vi "Subscr.Process Subscription Request.vi"(6 "Disable(Data2)":variant, 8 "error in (no error)":errorcluster, 9 "Request Info (Data1)":variant, 11 "Subscription in":refnum<class "Subscription.lvclass">) -> (0 "error out":errorcluster, 1 "SubScrReq":T1[](array[typedef]), 3 "Subscription out":refnum<class "Subscription.lvclass">)   [LabVIEW 2024, in "EQMF.lvlib" / "Subscription.lvlib" / "Subscription.lvclass"]
uses:
  Subscription.lvclass
  Subscr.Subscription Request Info.ctl
  Queues/Q.Element.ctl
  Subscription.lvclass/Subscription.ctl
  Queues/Queue Utils.lvlib
  Subscription.lvlib
panel:
  # "(For Ver/Debug)"
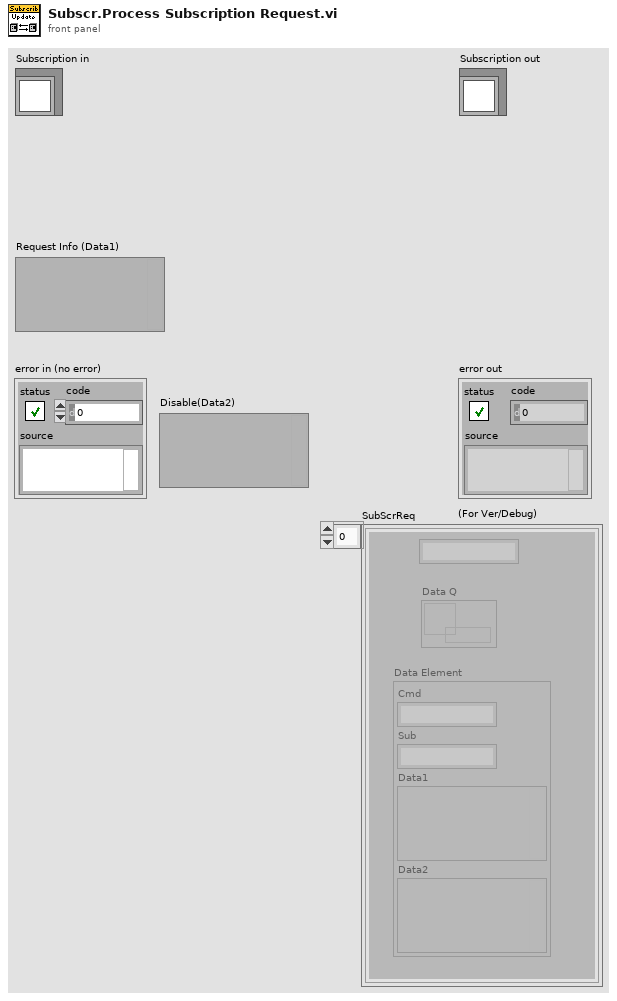
[diagram p1: front panel]
types:
  T1 = typedef "EQMF.lvlib/Subscription.lvlib/Subscr.Subscription Request Info.ctl" = cluster{"Name":string, "Data Q":refnum<queue>, "Data Element":T2}
  T2 = typedef "EQMF.lvlib/Queue Utils.lvlib/Q.Element.ctl" = cluster{"Cmd":string, "Sub":string, "Data1":variant, "Data2":variant}
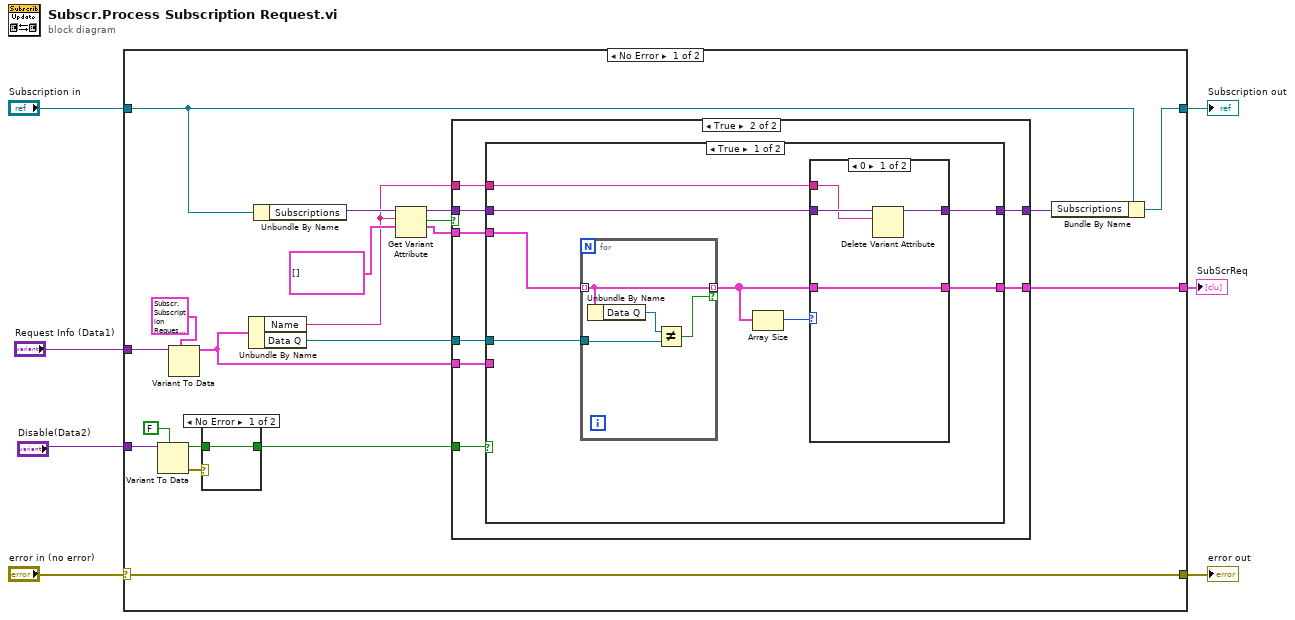
[diagram p0: block diagram]
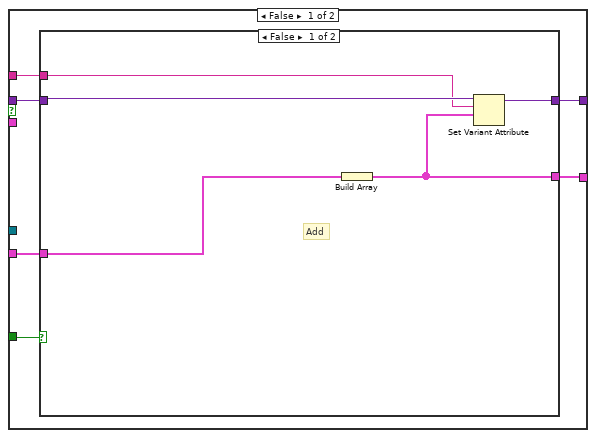
[diagram p2: hidden frame]
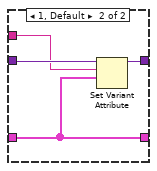
[diagram p4: hidden frame]
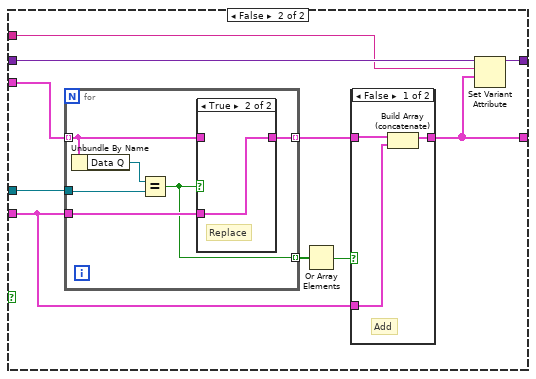
[diagram p5: hidden frame]
diagram:
  n1 = case shown="No Error" "error in (no error)" {
    selector: "error in (no error)" -> [w27 w92]
    tunnel: [w27 w92] -> w6
    tunnel: [w12 w91] -> w4
    tunnel: "Subscription in" -> [w11 w91]
    tunnel: "Request Info (Data1)" -> [w26 _]
    tunnel: "Disable(Data2)" -> [w24 _]
    tunnel: [w9 _] -> w1
    frame No Error {
      n2 = Variant To Data(type=FALSE, Variant=w24) -> (data=w21:bool, error out=w22:errorcluster)  [unwired: 1 in]
      n3 = Variant To Data(type=T1 {"Name"="", "Data Q"=refnum, "Data Element"={"Cmd"="", "Sub"="", "Data1"=variant, "Data2"=variant}} ("Event Destination"), Variant=w26) -> (data=w10:T1)  [unwired: 1 in, 1 out]
      n4 = case shown="No Error" w22 {
        tunnel: w21 -> [w90 _]
        tunnel: [w90 _] -> w14
        frame No Error {
        }
        frame Error {
        }
      }
      n5 = Unbundle By Name(w10) -> ("Name"=w8:string, "Data Q"=w15:refnum<queue>)
      n6 = Unbundle By Name(w11) -> ("Subscriptions"=w20:variant)
      n7 = Get Variant Attribute(Variant=w20, name=w8, default value (empty Variant)=T1[] []) -> (duplicate Variant=w17:variant, found=w18:bool, value=w16:T1[])  [unwired: 1 in, 1 out]
      n8 = case shown="True" w18 {
        tunnel: w17 -> [w32 w47]
        tunnel: w16 -> [_ w46]
        tunnel: w15 -> [_ w44]
        tunnel: w14 -> [w33 w45]
        tunnel: w8 -> [w30 w43]
        tunnel: [w31 w42] -> w13
        tunnel: w10 -> [w29 w41]
        tunnel: [w28 w40] -> w9
        frame False {
          n9 = case shown="False" w33 {
            tunnel: w32 -> [w37 w39]
            tunnel: [w38 w39] -> w31
            tunnel: w30 -> [w36 _]
            tunnel: w29 -> [w35 _]
            tunnel: [w34 _] -> w28
            frame False {
              # "Add"
              n10 = Build Array(w35) -> (w34:T1[])
              n11 = Set Variant Attribute(Variant=w37, name=w36, value=w34) -> (Variant out=w38:variant)  [unwired: 1 in, 2 out]
            }
            frame True {
              # "Do nothing.\nNo subscription to disable"
            }
          }
        }
        frame True {
          n12 = case shown="True" w45 {
            tunnel: w47 -> [w53 w75]
            tunnel: w46 -> [w55 w77]
            tunnel: w44 -> [w54 w76]
            tunnel: w43 -> [w51 w74]
            tunnel: [w50 w73] -> w42
            tunnel: w41 -> [_ w69]
            tunnel: [w48 w68] -> w40
            frame True {
              n13 = for {
                tunnel: w55 -> [w67] mode=indexing
                tunnel: w54 -> [w65]
                tunnel: [w67] -> w49 mode=indexing if=w64
                n14 = Unbundle By Name(w67) -> ("Data Q"=w66:refnum<queue>)
                n15 = Not Equal?(x=w66, y=w65) -> (x != y?=w64:bool)
              }
              n16 = Array Size(array=w49) -> (size(s)=w52:i32)
              n17 = case shown="0" w52 {
                tunnel: w53 -> [w59 w62]
                tunnel: w51 -> [w58 w61]
                tunnel: [w57 w63] -> w50
                tunnel: w49 -> [w56 w60]
                tunnel: [w56 w60] -> w48
                frame 0 {
                  n18 = Delete Variant Attribute(6:w58, 7:w59) -> (3:w57:variant)  [unwired: 1 in, 2 out]
                }
                frame 1, Default {
                  n19 = Set Variant Attribute(Variant=w62, name=w61, value=w60) -> (Variant out=w63:variant)  [unwired: 1 in, 2 out]
                }
              }
            }
            frame False {
              n20 = for {
                tunnel: w77 -> [w85] mode=indexing
                tunnel: w76 -> [w86]
                tunnel: [w83] -> w71 mode=indexing
                tunnel: w69 -> [w84]
                tunnel: [w82] -> w72 mode=indexing
                n21 = Unbundle By Name(w85) -> ("Data Q"=w87:refnum<queue>)
                n22 = Equal?(x=w87, y=w86) -> (x = y?=w82:bool)
                n23 = case shown="True" w82 {
                  tunnel: w85 -> [w88 _]
                  tunnel: w84 -> [_ w89]
                  tunnel: [w88 w89] -> w83
                  frame False {
                  }
                  frame True {
                    # "Replace"
                  }
                }
              }
              n24 = Or Array Elements(Boolean array=w72) -> (logical OR=w70:bool)
              n25 = case shown="False" w70 {
                tunnel: w71 -> [w80 w81]
                tunnel: w69 -> [w78 _]
                tunnel: [w79 w81] -> w68
                frame False {
                  # "Add"
                  n26 = Build Array (concatenate)(w80, w78) -> (w79:T1[])
                }
                frame True {
                }
              }
              n27 = Set Variant Attribute(Variant=w75, name=w74, value=w68) -> (Variant out=w73:variant)  [unwired: 1 in, 2 out]
            }
          }
        }
      }
      n28 = Bundle By Name(cluster=w11, "Subscriptions"=w13) -> (w12:refnum<class "Subscription.lvclass">)
    }
    frame Error {
    }
  }
  "error out" <- w6
  "Subscription out" <- w4
  "SubScrReq" <- w1
